vi "Pre Launch Init.vi"(11 "Datalogger Actor in":refnum<class "Datalogger Actor.lvclass">) -> (0 "error out":errorcluster, 3 "Datalogger Actor out":refnum<class "Datalogger Actor.lvclass">)   [LabVIEW 2018, in "Datalogger.lvlib" / "Datalogger Actor.lvclass"]
doc: "Sends a high priority message to it's self to notify the monitor that it's spawned. If it's in the runtime environment, this message is never sent, meaning the monitor will never spawn\n\nCopyright: MGI\nAuthored by: Derek Trepanier"
uses:
  Datalogger Actor.lvclass
  Data Record Control.ctl
  Datalogger Actor.lvclass/Datalogger Actor.ctl
  Actor Monitor/Actor/Monitored Actor.lvclass
types:
  T1 = typedef "Datalogger.lvlib/Datalogger Actor.lvclass/Data Record Control.ctl" = cluster{"Timestamp":string, "Sensor Name":string, "Data (string)":string, "Units":string}
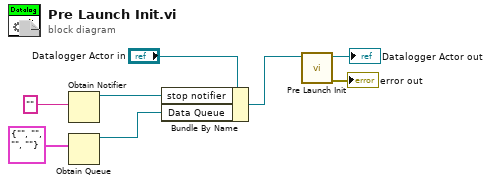
[diagram p0: block diagram]
diagram:
  n1 = Obtain Notifier(notification data type="") -> (notifier out=w4:refnum<notifier>)  [unwired: 3 in, 2 out]
  n2 = Obtain Queue(element data type=T1 {"Timestamp"="", "Sensor Name"="", "Data (string)"="", "Units"=""} ("Data Record")) -> (queue out=w1:refnum<queue>)  [unwired: 4 in, 2 out]
  n3 = Bundle By Name(cluster="Datalogger Actor in", "stop notifier"=w4, "Data Queue"=w1) -> (w3:refnum<class "Datalogger Actor.lvclass">)
  n4 = call-parent "Pre Launch Init.vi"("Monitored Actor in"=w3) -> ("error out"=→"error out":errorcluster, "Monitored Actor out"=→"Datalogger Actor out":refnum<class "Datalogger Actor.lvclass">)  [unwired: 9 in]
